vi "Input Demo 101.vi"() -> ()   [LabVIEW 2011]
doc: "This VI show how to use the basic functions in the Input Device palette. It will show information about all the joysticks, keyboards and mice attached to the system (number of axes, buttons, pov, and the name). It will also give the current information for the first joystick attached to the system (location and button pressed). The current information for the first keyboard and mouse will also be displayed."
uses:
  <vilib>/Utility/inputDevices.llb/closeJoystick.vi
  <vilib>/Utility/inputDevices.llb/closeKeyboard.vi
  <vilib>/Utility/inputDevices.llb/closeMouse.vi
  <vilib>/Utility/inputDevices.llb/joystickAcquire.vi
  <vilib>/Utility/inputDevices.llb/keyboardAcquire.vi
  <vilib>/Utility/inputDevices.llb/mouseAcquire.vi
panel:
  in  "Message":string="LabVIEW was unable\nto detect a joystick."
  in  "Button":string="Continue"
  out "Left Button Pressed":bool
  out "Axis Info":T1
  out "Mouse Info":T2(array[cluster])
  out "Keys Pressed":T3(array[ring])
  out "Key Info":T4(array[cluster])
  out "X-axis":i32
  out "Y-axis":i32
  out "Joystick Info":T5(array[cluster])
  out "POV 1":i32
  out "Button 1":bool
  in  "stop":bool
  # "JOYSTICKS"
  # "KEYBOARD/KEYPADS"
  # "MICE"
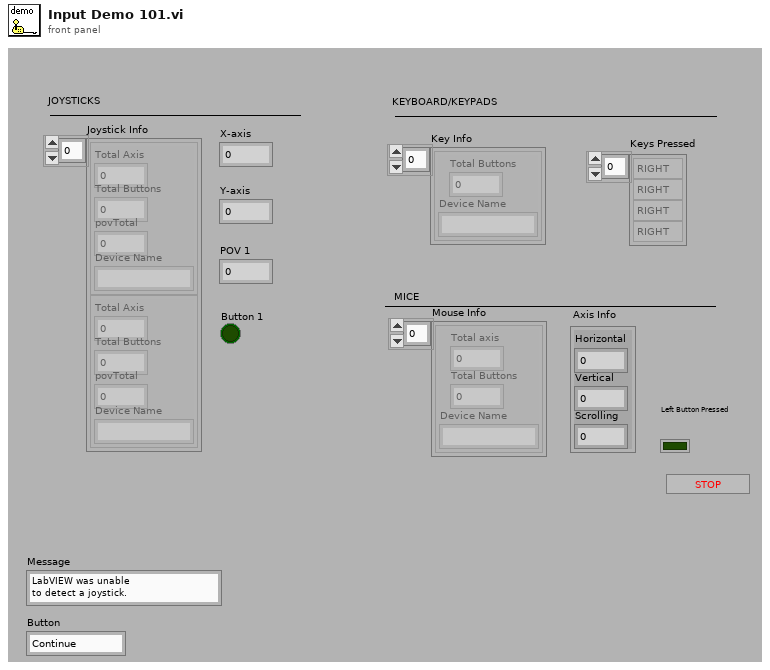
[diagram p1: front panel]
types:
  T1 = cluster{"Horizontal":i32, "Vertical":i32, "Scrolling":i32}
  T2 = cluster{"Total axis":u32, "Total Buttons":u32, "Device Name":string}[]
  T3 = enum16{"0", "1", "2", "3", "4", "5", "6", "7", "8", "9", "A", "B", "C", "D", "E", "F", "G", "H", "I", "J", "K", "L", "M", "N", "O", "P", "Q", "R", "S", "T", "U", "V", "W", "X", "Y", "Z", "F1", "F2", "F3", "F4", "F5", "F6", "F7", "F8", "F9", "F10", "F11", "F12", "F13", "F14", "F15", "ADD", "BACK", "BACKSLASH", "CAPITAL", "COMMA", "DECIMAL", "DELETE", "DIVIDE", "DOWN", "END", "EQUALS", "ESCAPE", "GRAVE (`)", "HOME", "INSERT", "LBRACKET", "LCONTROL", "LEFT", "L ALT", "LSHIFT", "LWIN", "MINUS", "MULTIPLY", "NEXT", "NUMLOCK", "NUMPAD_0", "NUMPAD_1", "NUMPAD_2", "NUMPAD_3", "NUMPAD_4", "NUMPAD_5", "NUMPAD_6", "NUMPAD_7", "NUMPAD_8", "NUMPAD_9", "PAUSE", "PERIOD", "PRIOR (PG UP)", "RBRACKET", "RCONTROL", "RETURN", "RIGHT", "R ALT", "RSHIFT", "RWIN", "SCROLL", "SEMICOLON", "SLASH", "SPACE", "SUBTRACT", "TAB", "UP", "ENTER (num pad)", "' (quote)"}[]
  T4 = cluster{"Total Buttons":u32, "Device Name":string}[]
  T5 = cluster{"Total Axis":u32, "Total Buttons":u32, "povTotal":u32, "Device Name":string}[]
  T6 = cluster{"axes total":u32, "buttons total":u32, "device name":string}[]
  T7 = cluster{"buttons total":u32, "device name":string}[]
  T8 = cluster{"axes total":u32, "buttons total":u32, "pov total":u32, "device name":string}[]
  T9 = cluster{"X axis":i32, "Y axis":i32, "Z axis":i32, "X axis rotation":i32, "Y axis rotation":i32, "Z axis rotation":i32, "U axis":i32, "V axis":i32}
  T10 = cluster{"button 1":bool, "button 2":bool, "button 3":bool, "button 4":bool, "button 5":bool, "button 6":bool, "button 7":bool, "button 8":bool, "button 9":bool, "button 10":bool, "button 11":bool, "button 12":bool, "button 13":bool, "button 14":bool, "button 15":bool, "button 16":bool, "button 17":bool, "button 18":bool, "button 19":bool, "button 20":bool, "button 21":bool, "button 22":bool, "button 23":bool, "button 24":bool, "button 25":bool, "button 26":bool, "button 27":bool, "button 28":bool, "button 29":bool, "button 30":bool, "button 31":bool, "button 32":bool}
  T11 = cluster{"pov 1":i32, "pov 2":i32, "pov 3":i32, "pov 4":i32}
  T12 = cluster{"button 1":bool, "button 2":bool, "button 3":bool, "button 4":bool}
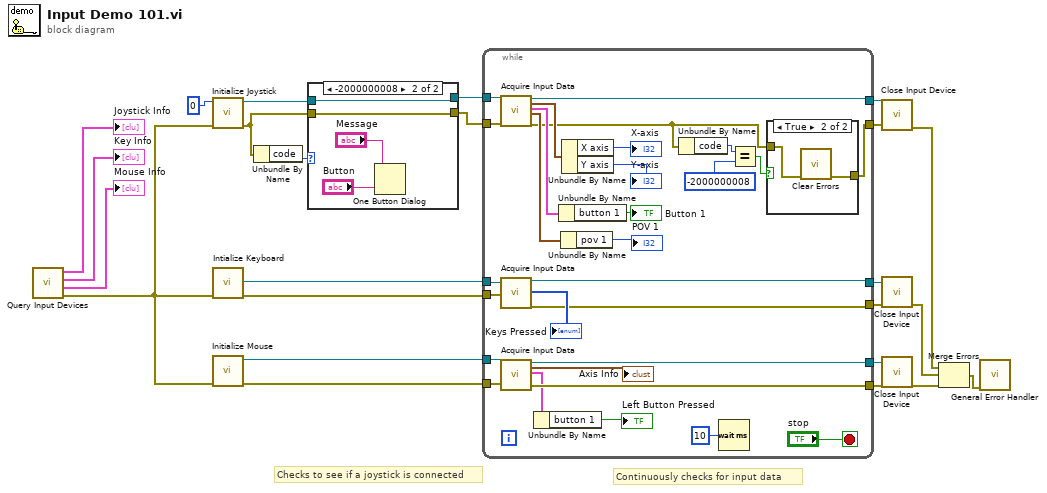
[diagram p0: block diagram]
diagram:
  # "Continuously checks for input data"
  # "Checks to see if a joystick is connected"
  n1 = call <vilib>:"Query Input Devices.vi"() -> ("error out"=w20:errorcluster, "mouse info"=→"Mouse Info":T6, "key info"=→"Key Info":T7, "joystick info"=→"Joystick Info":T8)  [unwired: 1 in, 7 out]
  n2 = call <vilib>:"Initialize Joystick.vi"("error in (no error)"=w20, "device index"=0) -> ("error out"=w3:errorcluster, "device ID"=w4:refnum<k1>)  [unwired: 8 out]
  n3 = call <vilib>:"Intialize Keyboard.vi"("error in (no error)"=w20) -> ("error out"=w22:errorcluster, "device ID"=w24:refnum<k1>)  [unwired: 9 out]
  n4 = call <vilib>:"Initialize Mouse.vi"("error in (no error)"=w20) -> ("error out"=w21:errorcluster, "device ID"=w23:refnum<k1>)  [unwired: 9 out]
  n5 = Unbundle By Name(w3) -> ("code"=w5:i32)
  n6 = case shown="-2000000008" w5 {
    tunnel: w3 -> [w26 w28]
    tunnel: [w26 w28] -> w2
    tunnel: w4 -> [w25 w27]
    tunnel: [w25 w27] -> w1
    frame 0, Default {
    }
    frame -2000000008 {
      n7 = One Button Dialog(message="Message", button name ("OK")="Button") -> ()  [unwired: 1 out]
    }
  }
  n8 = while {
    tunnel: [w47] -> w10
    tunnel: [w40] -> w11
    tunnel: [w48] -> w12
    tunnel: [w34] -> w14
    tunnel: w21 -> [w49]
    tunnel: w22 -> [w50]
    tunnel: w23 -> [w51]
    tunnel: [w42] -> w15
    tunnel: [w41] -> w13
    tunnel: w24 -> [w39]
    tunnel: w2 -> [w32]
    tunnel: w1 -> [w31]
    stop <- "stop" stop-if-true
    n9 = call-poly <vilib>:"Acquire Input Data.vi"("device ID"=w31, "error in (no error)"=w32) -> ("device ID"=w42:refnum<k1>, "axis info"=w59:T9, "button info"=w56:T10, "direction info"=w54:T11, "error out"=w33:errorcluster)  [unwired: 13 out]
    n10 = call-poly <vilib>:"Acquire Input Data.vi"("device ID"=w39, "error in (no error)"=w50) -> ("device ID"=w41:refnum<k1>, "keys pressed"=→"Keys Pressed":T3, "error out"=w48:errorcluster)  [unwired: 15 out]
    n11 = call-poly <vilib>:"Acquire Input Data.vi"("device ID"=w51, "error in (no error)"=w49) -> ("device ID"=w40:refnum<k1>, "axis info"=→"Axis Info":T1, "button info"=w46:T12, "error out"=w47:errorcluster)  [unwired: 1 in, 13 out]
    n12 = Unbundle By Name(w46) -> ("button 1"=→"Left Button Pressed":bool)
    n13 = Unbundle By Name(w56) -> ("button 1"=→"Button 1":bool)
    n14 = Unbundle By Name(w54) -> ("pov 1"=→"POV 1":i32)
    n15 = Unbundle By Name(w59) -> ("X axis"=→"X-axis":i32, "Y axis"=→"Y-axis":i32)
    n16 = Unbundle By Name(w33) -> ("code"=w37:i32)
    n17 = Wait (ms)(milliseconds to wait=u32 10) -> ()  [unwired: 1 out]
    n18 = Equal?(x=w37, y=-2000000008) -> (x = y?=w35:bool)
    n19 = case shown="True" w35 {
      tunnel: w33 -> [w60 w62]
      tunnel: [w60 w61] -> w34
      frame False {
      }
      frame True {
        n20 = call <vilib>:"Clear Errors.vi"("error in (no error)"=w62) -> ("error out"=w61:errorcluster)  [unwired: 6 out]
      }
    }
  }
  n21 = call-poly <vilib>:"Close Input Device.vi"("error in (no error)"=w14, "device ID"=w15) -> ("error out"=w6:errorcluster)  [unwired: 8 out]
  n22 = call-poly <vilib>:"Close Input Device.vi"("error in (no error)"=w12, "device ID"=w13) -> ("error out"=w7:errorcluster)  [unwired: 8 out]
  n23 = call-poly <vilib>:"Close Input Device.vi"("error in (no error)"=w10, "device ID"=w11) -> ("error out"=w9:errorcluster)  [unwired: 8 out]
  n24 = Merge Errors(w6, w7, w9) -> (w16:errorcluster)
  n25 = call <vilib>:"General Error Handler.vi"("error in (no error)"=w16) -> ()  [unwired: 1 in, 14 out]
